vi "GT Compare Pulse.vi"(7 "time":i16, 8 "error in (no error)":errorcluster caption="错误输入（无错误）", 9 "outputType":i16, 10 "level":i16, 11 "cardNum":i16) -> (0 "error out":errorcluster caption="错误输出", 3 "function return":i16)   [LabVIEW 2014, in "gts.lvlib"]
doc: "GT_API GT_ComparePulse(short cardNum,short level,short outputType,short time);"
uses:
  gts.lvlib
  gts.dll
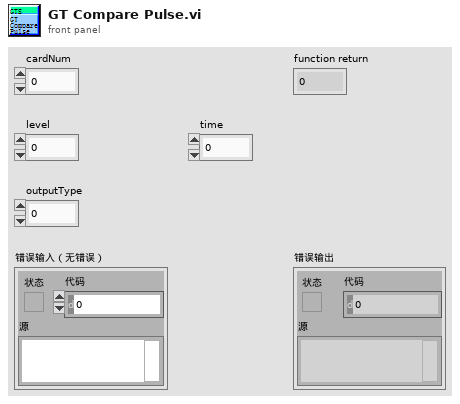
[diagram p1: front panel]
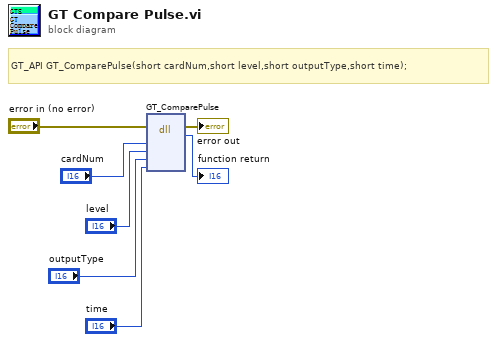
[diagram p0: block diagram]
diagram:
  # "GT_API GT_ComparePulse(short cardNum,short level,short outputType,short time);"
  n1 = dll-call lib="PTH2?abs D\t王淼清$控制卡常用功能例程(Labview)gts.*" fn="GT_ComparePulse"(error in="error in (no error)", "cardNum"="cardNum", "level"="level", "outputType"="outputType", "time"="time") -> (error out=→"error out":errorcluster, →"function return":i16)  [unwired: 6 in, 1 out]
